vi "手动调试界面.vi"() -> ()   [LabVIEW 2016, in "质控单元.lvlib"]
uses:
  <vilib>/Utility/miscctls.llb/LVPointTypeDef.ctl
panel:
  in  "CODCr水样":bool
  in  "CODMn水样":bool
  in  "总氮水样":bool
  in  "总磷水样":bool
  in  "氨氮水样":bool
  in  "CODCr加标":bool
  in  "CODMn加标":bool
  in  "氨氮加标":bool
  in  "总磷加标":bool
  in  "总氮加标":bool
  in  "总氮加标回收启动":bool
  in  "总氮停止":bool
  in  "总氮排液":bool
  in  "总氮调试":bool
  in  "CODCr加标回收启动":bool
  in  "CODCr停止":bool
  in  "CODCr排液":bool
  in  "CODCr调试":bool
  in  "CODMn加标回收启动":bool
  in  "CODMn停止":bool
  in  "CODMn排液":bool
  in  "CODMn调试":bool
  in  "总磷加标回收启动":bool
  in  "总磷停止":bool
  in  "总磷排液":bool
  in  "总磷调试":bool
  in  "氨氮加标回收启动":bool
  in  "氨氮停止":bool
  in  "氨氮排液":bool
  in  "氨氮调试":bool
  in  "关闭":bool
  # "手动调试界面"
  # "氨氮模块"
  # "总磷模块"
  # "总氮模块"
  # "CODMn模块"
  # "CODCr模块"
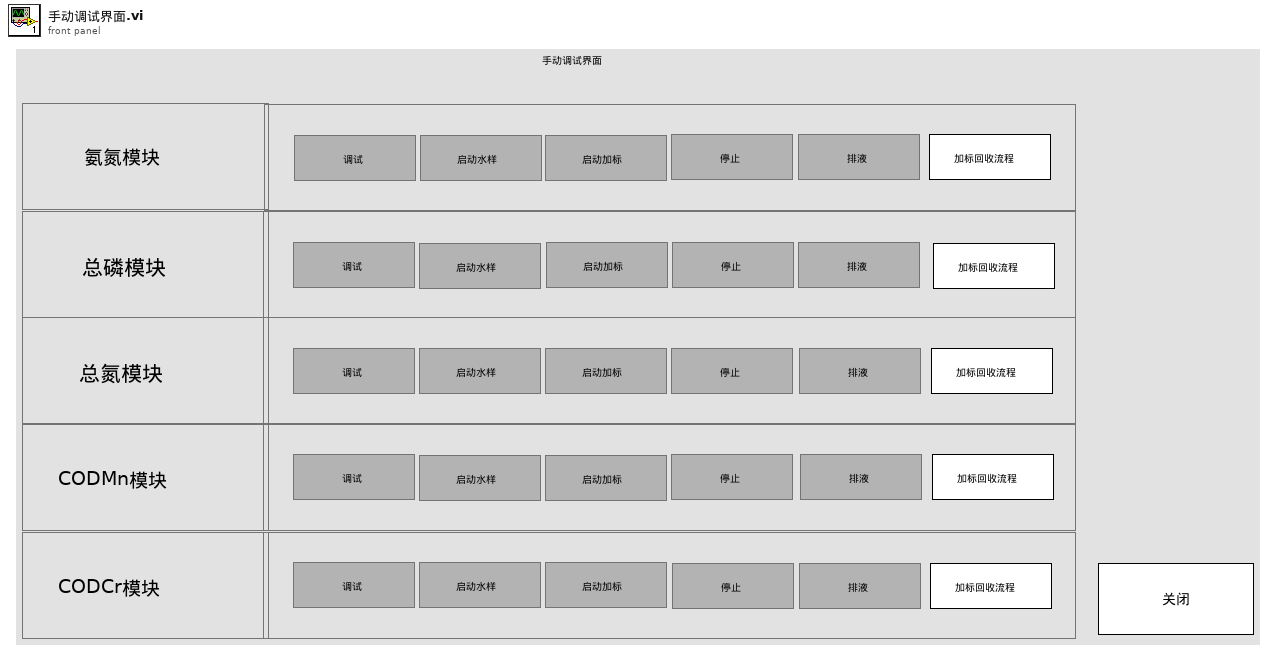
[diagram p1: front panel]
types:
  T1 = typedef "LVPointTypeDef.ctl" = cluster{"Horizontal":i16, "Vertical":i16}
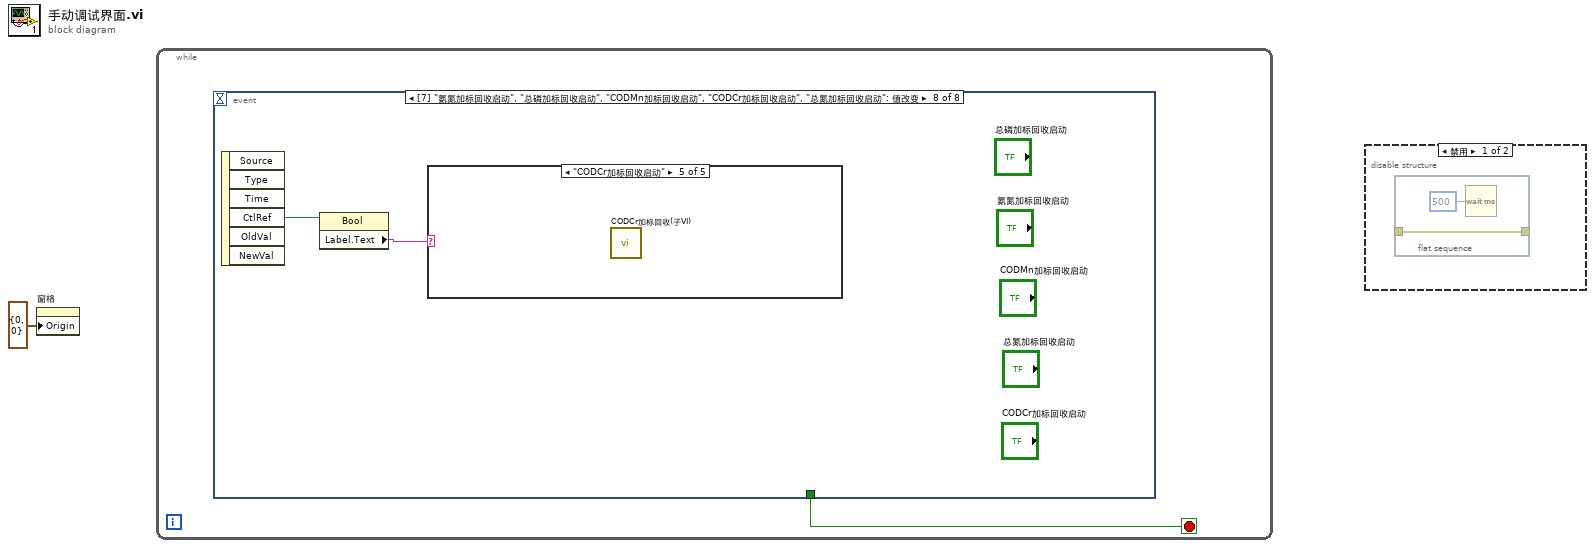
[diagram p0: block diagram]
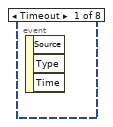
[diagram p3: hidden frame]
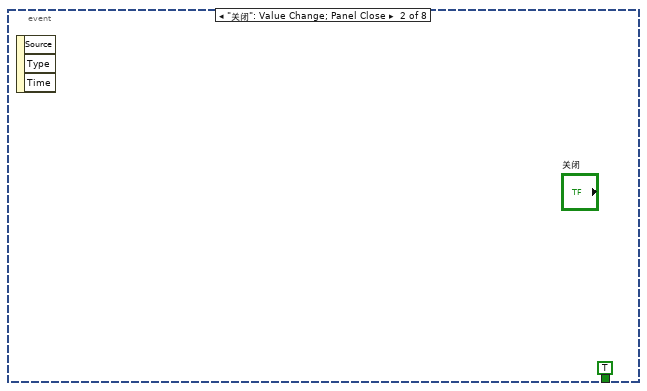
[diagram p4: hidden frame]
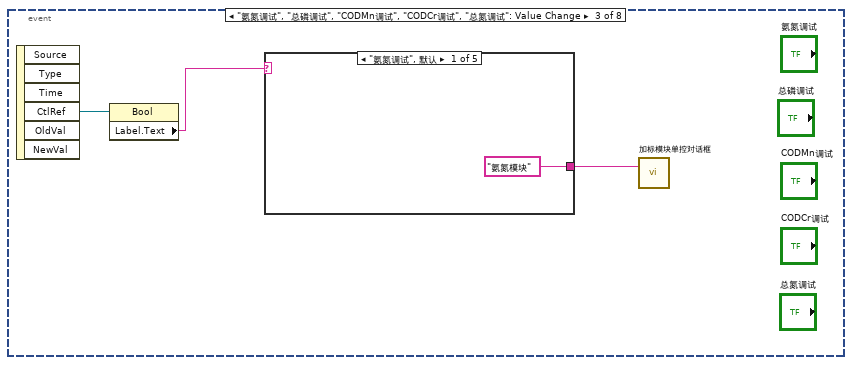
[diagram p5: hidden frame]
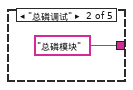
[diagram p6: hidden frame]
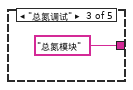
[diagram p7: hidden frame]
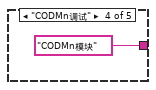
[diagram p8: hidden frame]
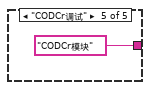
[diagram p9: hidden frame]
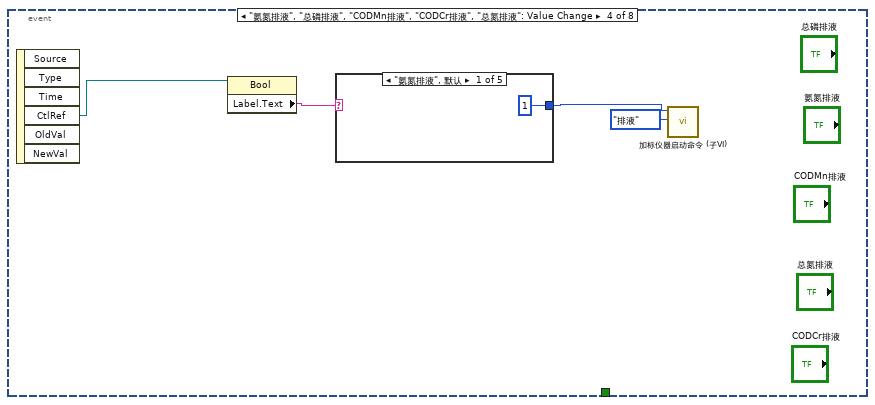
[diagram p10: hidden frame]
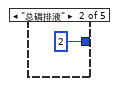
[diagram p11: hidden frame]
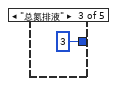
[diagram p12: hidden frame]
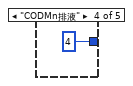
[diagram p13: hidden frame]
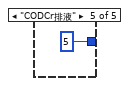
[diagram p14: hidden frame]
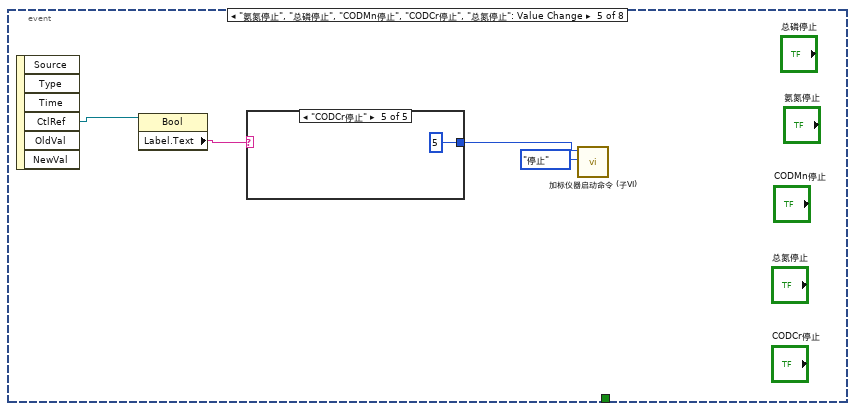
[diagram p15: hidden frame]
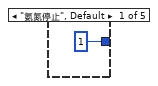
[diagram p16: hidden frame]
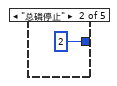
[diagram p17: hidden frame]
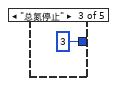
[diagram p18: hidden frame]
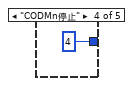
[diagram p19: hidden frame]
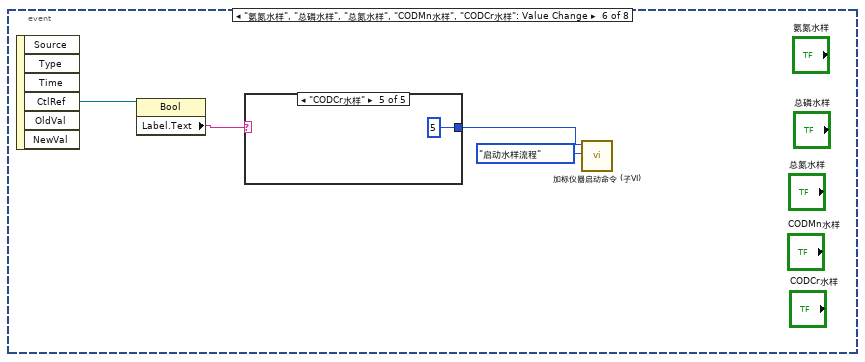
[diagram p20: hidden frame]
diagram:
  n1 = property on="窗格" class="Pane"("Origin"=T1 {"Horizontal"=0, "Vertical"=0} ("原点")) -> ()  [unwired: 2 in, 2 out]
  n2 = while {
    stop <- w2 stop-if-true
    n3 = event shown="[7] \"氨氮加标回收启动\", \"总磷加标回收启动\", \"CODMn加标回收启动\", \"CODCr加标回收启动\", \"总氮加标回收启动\": 值改变" {
      selector: _ -> [_ _ _ _ _ _ _ _]
      dyn-events: _ -> [_ _ _ _ _ _ _ _]
      timeout: _ -> [_ _ _ _ _ _ _ _]
      tunnel: [_ TRUE ("关闭") _ _ _ _ _ _] -> w2
      event Timeout {
        n4 = event-data() -> ()  [unwired: 1 in, 3 out]
      }
      event "关闭": Value Change; Panel Close {
        n5 = event-data() -> ()  [unwired: 1 in, 3 out]
      }
      event "氨氮调试", "总磷调试", "CODMn调试", "CODCr调试", "总氮调试": Value Change {
        n6 = event-data() -> ("CtlRef"=w5:refnum<vi>)  [unwired: 1 in, 5 out]
        n7 = property class="Bool"(reference=w5) -> ("Label.Text"=w4:string)  [unwired: 1 in, 2 out]
        n8 = case shown="\"氨氮调试\", 默认" w4 {
          tunnel: ["氨氮模块" ("标题") "总磷模块" ("标题") "总氮模块" ("标题") "CODMn模块" ("标题") "CODCr模块" ("标题")] -> w6
          frame "氨氮调试", Default {
          }
          frame "总磷调试" {
          }
          frame "总氮调试" {
          }
          frame "CODMn调试" {
          }
          frame "CODCr调试" {
          }
        }
        n9 = call "加标模块单控对话框.vi"("标题"=w6) -> ()  [unwired: 11 in]
      }
      event "氨氮排液", "总磷排液", "CODMn排液", "CODCr排液", "总氮排液": Value Change {
        n10 = event-data() -> ("CtlRef"=w14:refnum<vi>)  [unwired: 1 in, 5 out]
        n11 = property class="Bool"(reference=w14) -> ("Label.Text"=w15:string)  [unwired: 1 in, 2 out]
        n12 = case shown="\"氨氮排液\", 默认" w15 {
          tunnel: [u8 1 ("Slave ID") u8 2 ("Slave ID") u8 3 ("Slave ID") u8 4 ("Slave ID") u8 5 ("Slave ID")] -> w12
          frame "氨氮排液", Default {
          }
          frame "总磷排液" {
          }
          frame "总氮排液" {
          }
          frame "CODMn排液" {
          }
          frame "CODCr排液" {
          }
        }
        n13 = call "加标仪器启动命令 (子VI).vi"("启动命令"=enum16{"启动水样流程", "启动加标流程", "排液", "停止"}."排液", "仪器"=w12) -> ()  [unwired: 9 in, 1 out]
      }
      event "氨氮停止", "总磷停止", "CODMn停止", "CODCr停止", "总氮停止": Value Change {
        n14 = event-data() -> ("CtlRef"=w23:refnum<vi>)  [unwired: 1 in, 5 out]
        n15 = property class="Bool"(reference=w23) -> ("Label.Text"=w24:string)  [unwired: 1 in, 2 out]
        n16 = case shown="\"CODCr停止\"" w24 {
          tunnel: [u8 1 ("Slave ID") u8 2 ("Slave ID") u8 3 ("Slave ID") u8 4 ("Slave ID") u8 5 ("Slave ID")] -> w21
          frame "氨氮停止", Default {
          }
          frame "总磷停止" {
          }
          frame "总氮停止" {
          }
          frame "CODMn停止" {
          }
          frame "CODCr停止" {
          }
        }
        n17 = call "加标仪器启动命令 (子VI).vi"("启动命令"=enum16{"启动水样流程", "启动加标流程", "排液", "停止"}."停止", "仪器"=w21) -> ()  [unwired: 9 in, 1 out]
      }
      event "氨氮水样", "总磷水样", "总氮水样", "CODMn水样", "CODCr水样": Value Change {
        n18 = event-data() -> ("CtlRef"=w32:refnum<vi>)  [unwired: 1 in, 5 out]
        n19 = property class="Bool"(reference=w32) -> ("Label.Text"=w33:string)  [unwired: 1 in, 2 out]
        n20 = case shown="\"CODCr水样\"" w33 {
          tunnel: [u8 1 ("Slave ID") u8 2 ("Slave ID") u8 3 ("Slave ID") u8 4 ("Slave ID") u8 5 ("Slave ID")] -> w30
          frame "氨氮水样", Default {
          }
          frame "总磷水样" {
          }
          frame "总氮水样" {
          }
          frame "CODMn水样" {
          }
          frame "CODCr水样" {
          }
        }
        n21 = call "加标仪器启动命令 (子VI).vi"("启动命令"=enum16{"启动水样流程", "启动加标流程", "排液", "停止"}."启动水样流程", "仪器"=w30) -> ()  [unwired: 9 in, 1 out]
      }
      event "氨氮加标", "总磷加标", "总氮加标", "CODMn加标", "CODCr加标": Value Change {
        n22 = event-data() -> ("CtlRef"=w46:refnum<vi>)  [unwired: 1 in, 5 out]
        n23 = property class="Bool"(reference=w46) -> ("Label.Text"=w47:string)  [unwired: 1 in, 2 out]
        n24 = case shown="\"CODCr加标\"" w47 {
          tunnel: [u8 1 ("Slave ID") u8 2 ("Slave ID") u8 3 ("Slave ID") u8 4 ("Slave ID") u8 5 ("Slave ID")] -> w43
          tunnel: [w48 w50 w52 w54 w56] -> w40
          frame "氨氮加标", Default {
            n25 = global read "加标回收状态全局变量.vi" "氨氮加标体积"() -> (w48:dbl)
          }
          frame "总磷加标" {
            n26 = global read "加标回收状态全局变量.vi" "总磷加标体积"() -> (w50:dbl)
          }
          frame "总氮加标" {
            n27 = global read "加标回收状态全局变量.vi" "总氮加标体积"() -> (w52:dbl)
          }
          frame "CODMn加标" {
            n28 = global read "加标回收状态全局变量.vi" "CODMn加标体积"() -> (w54:dbl)
          }
          frame "CODCr加标" {
            n29 = global read "加标回收状态全局变量.vi" "CODCr加标体积"() -> (w56:dbl)
          }
        }
        n30 = Build Array(w40) -> (w41:dbl[])
        n31 = call "浮点转DCBA整形ZK.vi"("浮点数"=w41) -> ("DCBA整形输出"=w39:u16[])  [unwired: 10 in]
        n32 = call "写入参数.vi"("values"=w39, "starting address"=u16 5, "Slave ID"=w43) -> ("error out"=w42:errorcluster)  [unwired: 8 in]
        n33 = call "加标仪器启动命令 (子VI).vi"("Error in"=w42, "启动命令"=enum16{"启动水样流程", "启动加标流程", "排液", "停止"}."启动加标流程", "仪器"=w43) -> ()  [unwired: 8 in, 1 out]
      }
      event "氨氮加标回收启动", "总磷加标回收启动", "CODMn加标回收启动", "CODCr加标回收启动", "总氮加标回收启动": Value Change {
        n34 = event-data() -> ("CtlRef"=w58:refnum<vi>)  [unwired: 1 in, 5 out]
        n35 = property class="Bool"(reference=w58) -> ("Label.Text"=w59:string)  [unwired: 1 in, 2 out]
        n36 = case shown="\"CODCr加标回收启动\"" w59 {
          frame "氨氮加标回收启动", Default {
            n37 = call "氨氮加标回收 (子VI).vi"() -> ()  [unwired: 12 in]
          }
          frame "总磷加标回收启动" {
            n38 = call "总磷加标回收 (子VI).vi"() -> ()  [unwired: 12 in]
          }
          frame "总氮加标回收启动" {
            n39 = call "总氮加标回收 (子VI).vi"() -> ()  [unwired: 12 in]
          }
          frame "CODMn加标回收启动" {
            n40 = call "CODMn加标回收(子VI).vi"() -> ()  [unwired: 12 in]
          }
          frame "CODCr加标回收启动" {
            n41 = call "CODCr加标回收(子VI).vi"() -> ()  [unwired: 12 in]
          }
        }
      }
    }
  }
  n42 = disable-structure shown="禁用" {
    frame Disabled {
      n43 = flat-sequence {
        tunnel: _ -> [w60]
        tunnel: [w60] -> _
        frame #0 {
          n44 = Wait (ms)(milliseconds to wait=u32 500 ("等待时间（毫秒）")) -> ()  [unwired: 1 out]
        }
      }
    }
    frame Enabled {
    }
  }
